vi "Keep_Frames.vi"(2 "old list":string[][](array[string]), 3 "list":string[][](array[string])) -> (0 "kept indices":i32[](array[numeric]), 1 "kept frames":string[](array[string]))   [LabVIEW 2012]
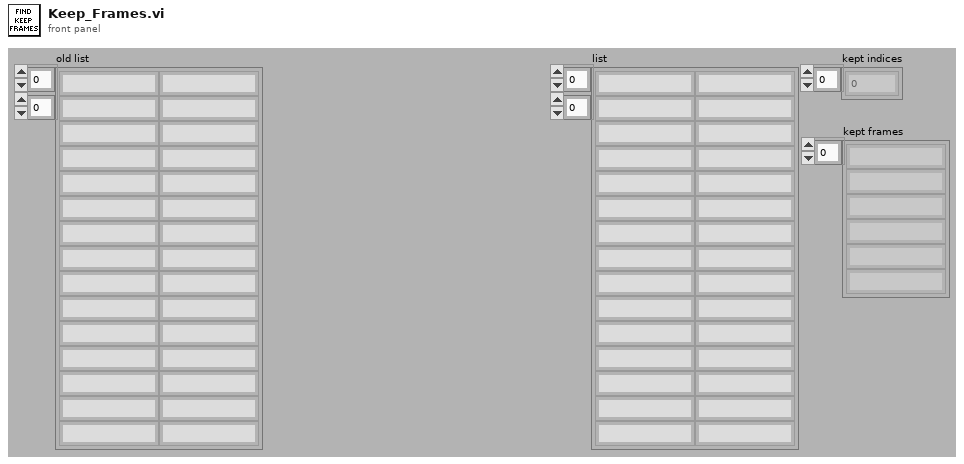
[diagram p1: front panel]
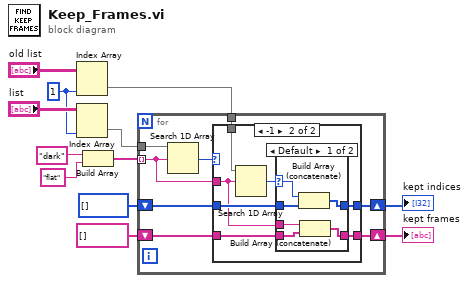
[diagram p0: block diagram]
diagram:
  w4 = 1 ("disabled index (col)")
  n1 = Index Array(array="old list", index (col)=w4) -> (element=w5:string[])  [unwired: 1 in]
  n2 = Index Array(array="list", index (col)=w4) -> (element=w6:string[])  [unwired: 1 in]
  n3 = Build Array("dark" ("element"), "flat" ("element")) -> (w12:string[])
  n4 = for {
    tunnel: w6 -> [w13]
    tunnel: w12 -> [w19] mode=indexing
    tunnel: w5 -> [w20]
    shift-right: [w16] -> w3
    shift-left: i32[] [] -> [w17]
    shift-right: [w14] -> w9
    shift-left: string[] [] -> [w15]
    n5 = Search 1D Array(1D array=w13, element=w19) -> (index of element=w18:i32)  [unwired: 1 in]
    n6 = case shown="-1" w18 {
      tunnel: w20 -> [_ w24]
      tunnel: w19 -> [_ w23]
      tunnel: w17 -> [w22 w28]
      tunnel: [w22 w27] -> w16
      tunnel: w15 -> [w21 w26]
      tunnel: [w21 w25] -> w14
      frame Default {
      }
      frame -1 {
        n7 = Search 1D Array(1D array=w24, element=w23) -> (index of element=w29:i32)  [unwired: 1 in]
        n8 = case shown="Default" w29 {
          selector: w29 -> [w34 _]
          tunnel: w28 -> [w35 w37]
          tunnel: [w33 w37] -> w27
          tunnel: w23 -> [w32 _]
          tunnel: w26 -> [w31 w36]
          tunnel: [w30 w36] -> w25
          frame Default {
            n9 = Build Array (concatenate)(w34, w35) -> (w33:i32[])
            n10 = Build Array (concatenate)(w32, w31) -> (w30:string[])
          }
          frame -1 {
          }
        }
      }
    }
  }
  "kept frames" <- w9
  "kept indices" <- w3
